vi "uObserver_Publish_Event.vi"(8 "error in (no error)":errorcluster, 10 "uMsg":refnum<class "uMsg.lvclass">, 11 "uObserver in":refnum<class "uObserver.lvclass">) -> (0 "error out":errorcluster, 3 "uObserver out":refnum<class "uObserver.lvclass">)   [LabVIEW 2023, in "uLib.lvlib" / "uObserver.lvclass"]
doc: "Publish an event to the observed broker conforming to the Observer's publishing policy.\nFor optimal performance in high-throughput streaming applications, make sure to set a valid timestamp when creating the message to be published."
uses:
  uObserver.lvclass
  uMsg/uMsg/uMsg.lvclass
  uObserver.lvclass/uObserver.ctl
  uClient/uClient_Publisher/uClient_Publisher.lvclass/uClient_Publisher.ctl
  uMsg/uMsg/uMsg.lvclass/uMsg.ctl
  uData/uData/uData.lvclass/uData.ctl
  uData/uData/Set Tag.vi
  uMsg/uMsg/uMsg Update Timestamp.vi
  uMsg/uMsg/uMsg Rename CMD.vi
  uMsg/uMsg/uMsg Get CMD.vi
  uMsg/uMsg/Write Payload.vi
  uMsg/uMsg/uMsg Create.vi
  uData/uData/Condition Tag Name.vi
  uData/uData/Blank Key Reserved String.vi
  uData/uData/uData.lvclass
  uTransport/uTransport/uTransport.lvclass
  uStringManipulation/uStringManipulation/uStringManipulation.lvclass
  uClient/uClient_Publisher/uClient_Publisher.lvclass
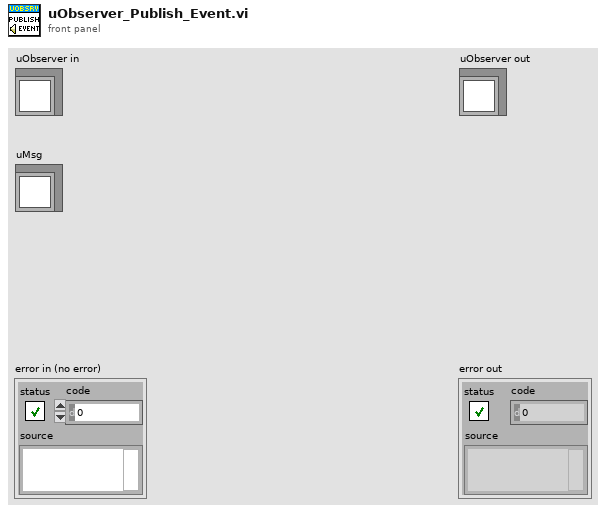
[diagram p1: front panel]
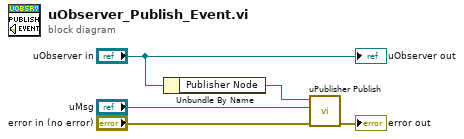
[diagram p0: block diagram]
diagram:
  n1 = Unbundle By Name("uObserver in") -> ("Publisher Node"=w1:refnum<class "uClient_Publisher.lvclass">)
  n2 = call "uPublisher Publish.vi"("error in (no error)"="error in (no error)", "uMsg"="uMsg", "uClient_Publisher in"=w1) -> ("error out"=→"error out":errorcluster)  [unwired: 7 in, 1 out]
  "uObserver out" <- "uObserver in"
